vi "Append Image to Report (string).vi"(0 "report in":refnum<class "NI_report.lvclass">, 1 "alignment (default)":T1, 2 "MS Office parameters":T2, 7 "path or URL of image":string, 9 "caption or alternative string":string, 11 "error in (no error)":errorcluster) -> (4 "report out":refnum<class "NI_report.lvclass">, 8 "start out (Word)":i32, 10 "end out (Word)":i32, 15 "error out":errorcluster)   [LabVIEW 2020, in "NI_report.lvclass"]
doc: "For an HTML report, the VI embeds a link to an image into the report. For a standard report, the VI appends the image from a file. You can wire either a path to the image or a string that contains the image URL to this polymorphic VI. The data type you wire to the <B>path or URL of image</B> input determines the polymorphic instance to use."
uses:
  NI_report.lvclass
  HTML Report Image Alignment.ctl
  NI_ReportGenerationCore.lvlib
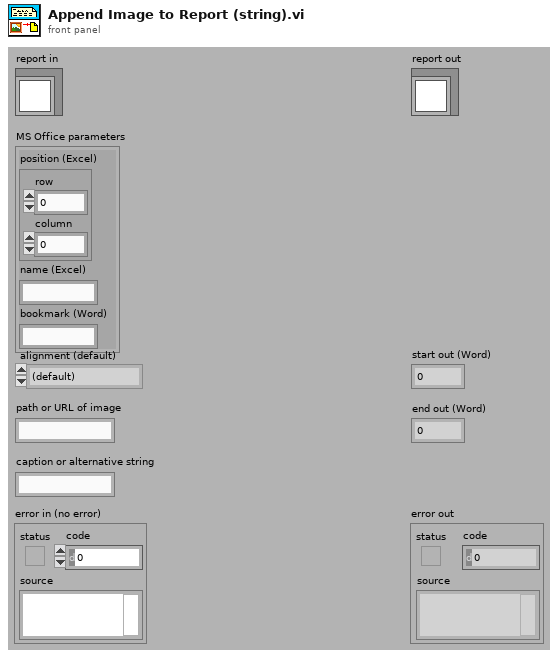
[diagram p1: front panel]
types:
  T1 = typedef "NI_ReportGenerationCore.lvlib/HTML Report Image Alignment.ctl" = enum16{"(default)", "LEFT", "RIGHT", "TOP", "TEXTTOP", "MIDDLE", "ABSMIDDLE", "BASELINE", "BOTTOM", "ABSBOTTOM"}
  T2 = cluster{"position (Excel)":cluster{"row":i32, "column":i32}, "name (Excel)":string, "bookmark (Word)":string}
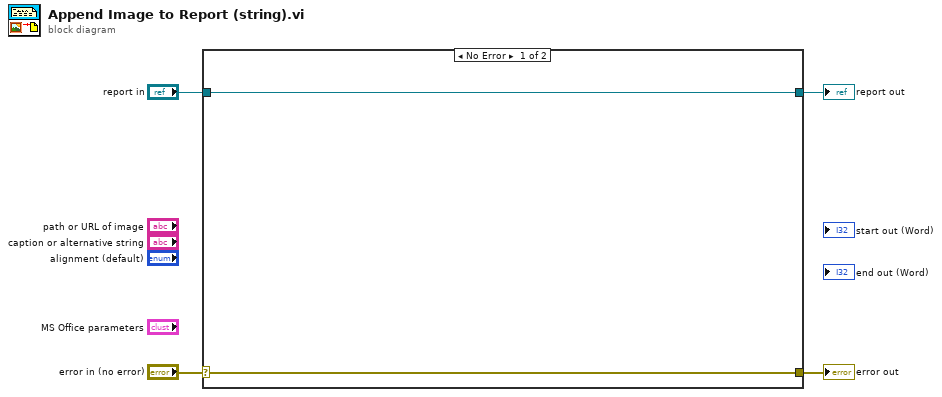
[diagram p0: block diagram]
diagram:
  n1 = case shown="No Error" "error in (no error)" {
    selector: "error in (no error)" -> [w5 w8]
    tunnel: [w5 w8] -> w3
    tunnel: [w6 w7] -> w1
    tunnel: "report in" -> [w6 w7]
    frame No Error {
    }
    frame Error {
    }
  }
  "error out" <- w3
  "report out" <- w1
